vi "Claps.vi"(8 "Objects":T1[](array[typedef]) {"Aspect Ratio" format="%.2f"; "Orientation" format="%.2f"; "Area" format="%.2f"; "Object Center"."Y" format="%.2f"; "Object Center"."X" format="%.2f"}) -> (0 "Start":bool)   [LabVIEW 2015]
uses:
  TypeDefs Host/Object Info.ctl
  TypeDefs Host/Open Audio FGV Enum.ctl
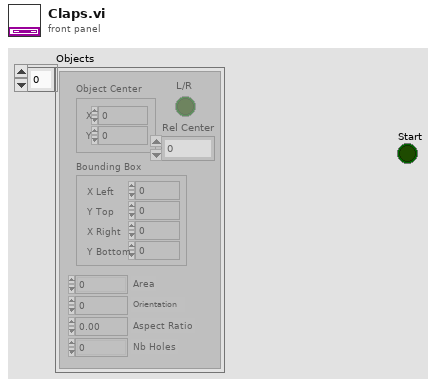
[diagram p1: front panel]
types:
  T1 = typedef "Object Info.ctl" = cluster{"Object Center":cluster{"X":u16, "Y":u16}, "Bounding Box":cluster{"X Left":u16, "Y Top":u16, "X Right":u16, "Y Bottom":u16}, "Area":u16, "Orientation":u16, "Aspect Ratio":sgl, "Nb Holes":u16, "L/R":bool, "Rel Center":u16}
  T2 = typedef "Open Audio FGV Enum.ctl" = enum16{"Get", "Set"}
  T3 = cluster{"X Left":u16, "Y Top":u16, "X Right":u16, "Y Bottom":u16}
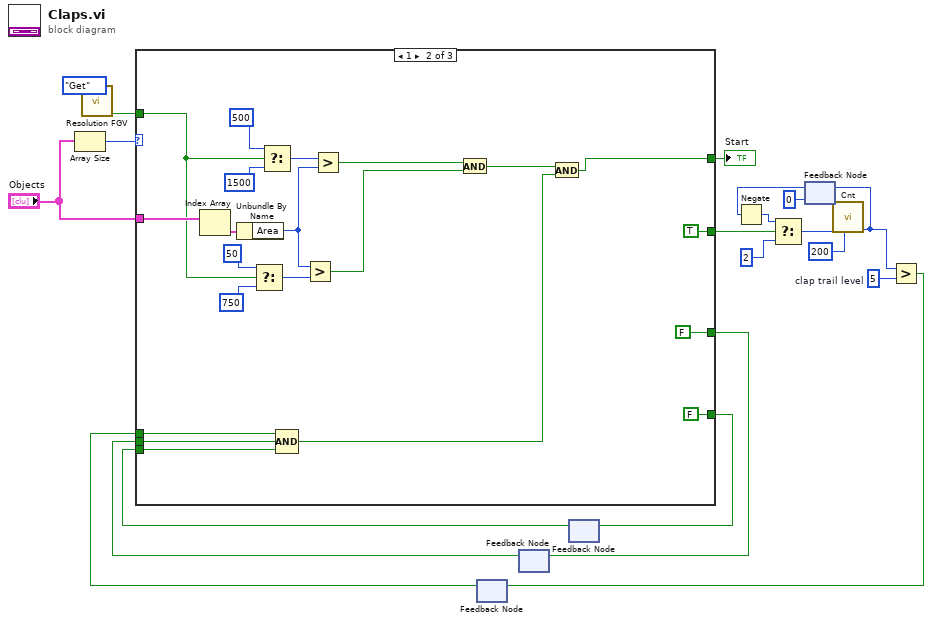
[diagram p0: block diagram]
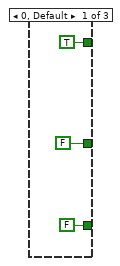
[diagram p2: hidden frame]
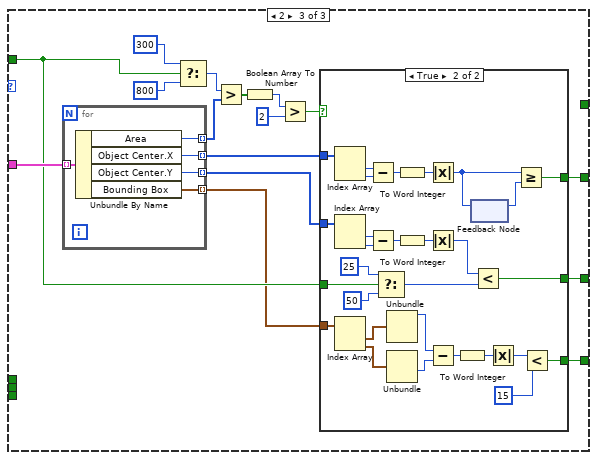
[diagram p3: hidden frame]
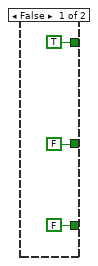
[diagram p4: hidden frame]
diagram:
  w8 = 5  # clap trail level
  n1 = Array Size(array="Objects") -> (size(s)=w20:i32)
  n2 = call "Resolution FGV.vi"("Command"=Open_Audio_FGV_Enum."Get") -> ("L/T?"=w6:bool)  [unwired: 10 in]
  n3 = feedback #1() -> (w11:bool)  [unwired: 1 in]
  n4 = feedback #2() -> (w4:bool)  [unwired: 1 in]
  n5 = feedback #3() -> (w3:bool)  [unwired: 1 in]
  n6 = case shown="1" w20 {
    tunnel: "Objects" -> [_ w43 w60]
    tunnel: [TRUE TRUE w53] -> w12
    tunnel: w11 -> [_ w26 _]
    tunnel: [_ w39 _] -> w10
    tunnel: w6 -> [_ w34 w48]
    tunnel: [FALSE FALSE w49] -> w5
    tunnel: w4 -> [_ w25 _]
    tunnel: [FALSE FALSE w45] -> w2
    tunnel: w3 -> [_ w24 _]
    frame 0, Default {
    }
    frame 1 {
      n7 = Index Array(array=w43) -> (element=w42:T1)  [unwired: 1 in]
      n8 = Unbundle By Name(w42) -> ("Area"=w40:u16)
      n9 = Select(t=u16 50 ("y"), s=w34, f=u16 750 ("y")) -> (s? t:f=w37:u16)
      n10 = Select(t=u16 500 ("x"), s=w34, f=u16 1500 ("x")) -> (s? t:f=w38:u16)
      n11 = Compound Arithmetic op=AND(w26, w25, w24) -> (w30:bool)
      n12 = Greater?(x=w40, y=w37) -> (0:w27:bool)
      n13 = Greater?(x=w38, y=w40) -> (0:w28:bool)
      n14 = And(x=w28, y=w27) -> (x .and. y?=w41:bool)
      n15 = And(x=w41, y=w30) -> (x .and. y?=w39:bool)
    }
    frame 2 {
      n16 = for {
        tunnel: w60 -> [w97] mode=indexing
        tunnel: [w96] -> w59 mode=indexing
        tunnel: [w95] -> w54 mode=indexing
        tunnel: [w94] -> w47 mode=indexing
        tunnel: [w93] -> w46 mode=indexing
        n17 = Unbundle By Name(w97) -> ("Area"=w96:u16, "Object Center.X"=w95:u16, "Object Center.Y"=w94:u16, "Bounding Box"=w93:T3)
      }
      n18 = Select(t=u16 300 ("Area"), s=w48, f=u16 800 ("Area")) -> (s? t:f=w50:u16)
      n19 = Greater?(x=w50, y=w59) -> (0:w58:bool[])
      n20 = Boolean Array To Number(Boolean array=w58) -> (number=w57:u32)
      n21 = Greater?(x=w57, y=u32 2) -> (0:w55:bool)
      n22 = case shown="True" w55 {
        tunnel: w54 -> [_ w92]
        tunnel: [TRUE w86] -> w53
        tunnel: [FALSE w84] -> w49
        tunnel: w48 -> [_ w85]
        tunnel: w47 -> [_ w79]
        tunnel: w46 -> [_ w73]
        tunnel: [FALSE w64] -> w45
        frame False {
        }
        frame True {
          n23 = Index Array(array=w92) -> (element #1=w91:u16, element #2=w90:u16)  [unwired: 2 in]
          n24 = Index Array(array=w79) -> (element #1=w76:u16, element #2=w75:u16)  [unwired: 2 in]
          n25 = Index Array(array=w73) -> (element #1=w72:T3, element #2=w71:T3)  [unwired: 2 in]
          n26 = Subtract(x=w91, y=w90) -> (x-y=w89:u16)
          n27 = Subtract(x=w76, y=w75) -> (x-y=w77:u16)
          n28 = Select(t=i16 25 ("abs(x)"), s=w85, f=i16 50 ("abs(x)")) -> (s? t:f=w82:i16)
          n29 = Unbundle(w72) -> ("X Left"=w68:u16)  [unwired: 3 out]
          n30 = Unbundle(w71) -> ("X Right"=w67:u16)  [unwired: 3 out]
          n31 = To Word Integer(number=w89) -> (16bit integer=w88:i16)
          n32 = To Word Integer(number=w77) -> (16bit integer=w78:i16)
          n33 = Absolute Value(x=w88) -> (abs(x)=w83:i16)
          n34 = Absolute Value(x=w78) -> (abs(x)=w74:i16)
          n35 = Subtract(x=w68, y=w67) -> (x-y=w69:u16)
          n36 = To Word Integer(number=w69) -> (16bit integer=w70:i16)
          n37 = feedback-in #4(w83) -> ()
          n38 = feedback #4() -> (w87:i16)  [unwired: 1 in]
          n39 = Less?(x=w74, y=w82) -> (x < y?=w84:bool)
          n40 = Absolute Value(x=w70) -> (abs(x)=w66:i16)
          n41 = Greater Or Equal?(x=w83, y=w87) -> (x >= y?=w86:bool)
          n42 = Less?(x=w66, y=i16 15) -> (x < y?=w64:bool)
        }
      }
    }
  }
  "Start" <- w10
  n43 = feedback-in #2(w5) -> ()
  n44 = feedback-in #3(w2) -> ()
  n45 = feedback #5(0 ("i")) -> (w13:i32)
  n46 = Negate(x=w13) -> (-x=w14:i32)
  n47 = Select(t=w14, s=w12, f=2) -> (s? t:f=w15:i32)
  n48 = call "Cnt.vi"("n-1"=200, "inc"=w15) -> ("i"=w9:i32)  [unwired: 8 in, 1 out]
  n49 = feedback-in #5(w9) -> ()
  n50 = Greater?(x=w9, y=w8) -> (0:w1:bool)
  n51 = feedback-in #1(w1) -> ()
